vi "Create Fake Session Factory.vi"(8 "error in":errorcluster, 9 "service class":string, 10 "provided interface":string, 11 "instrument type id":string="fake_instrument_type") -> (0 "error out":errorcluster, 3 "fake session factory out":refnum<class "Fake Session Factory.lvclass">)   [LabVIEW 2020, in "MeasurementServerTests.lvlib" / "Fake Session Factory.lvclass"]
uses:
  Fake Session Factory.lvclass
  Call Recorder Action.ctl
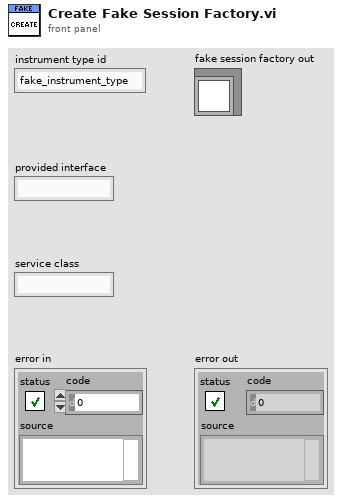
[diagram p1: front panel]
types:
  T1 = typedef "MeasurementServerTests.lvlib/Fake Session Factory.lvclass/Call Recorder Action.ctl" = enum16{"Initialize", "Read Values", "Record Initialize-Initialize", "Record Initialize-Attach", "Record Close-Close", "Record Close-Detach"}
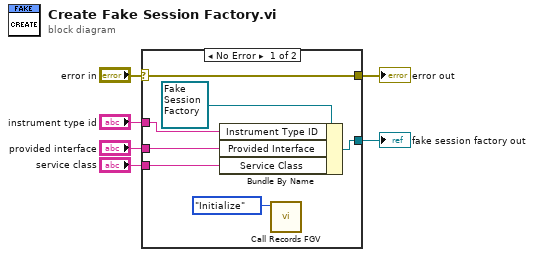
[diagram p0: block diagram]
diagram:
  n1 = case shown="No Error" "error in" {
    selector: "error in" -> [w13 w14]
    tunnel: [w13 w14] -> w5
    tunnel: [w11 _] -> w4
    tunnel: "instrument type id" -> [w10 _]
    tunnel: "provided interface" -> [w9 _]
    tunnel: "service class" -> [w7 _]
    frame No Error {
      n2 = Bundle By Name(cluster=refnum<class "Fake Session Factory.lvclass"> refnum ("fake instrument out"), "Instrument Type ID"=w10, "Provided Interface"=w9, "Service Class"=w7) -> (w11:refnum<class "Fake Session Factory.lvclass">)
      n3 = call "Call Records FGV.vi"("call recorder action"=Call_Recorder_Action."Initialize" ("Call Recorder Action")) -> ()  [unwired: 7 in, 4 out]
    }
    frame Error {
    }
  }
  "error out" <- w5
  "fake session factory out" <- w4
